vi "OE1311&OE1351_Configure Ref Phase.vi"(7 "OE1300_Configure Ref Phase":T1={"Reference Source"=0, "Internal Frequency(Hz)"=1000.0, "Phase  (degree)"=0.0, "External Ref Trigger"=0, "Instrument Mode "=4} {"Instrument Mode" items=["OE1311"=3, "OE1351"=4, "OE1301"=5]; "External Ref Trigger" items=["TTL Rising Edge", "TTL Fallling Edge", "Sine Zero Crossing"]; "Phase  (degree)" min=-180.0 max=180.0 format="%#.2g"; "Internal Frequency(Hz)" min=0.001 max=1002000.0 format="%#.3f"; "Reference Source" items=["External", "Internal", "Self"]}, 8 "Error in (no error)":errorcluster caption="error out（no error）", 9 "Remote Mode":u16(ring)=1 items=["RS232"=1, "Ethernet"=3], 10 "Connection ID in":refnum<k5>, 11 "VISA resource name":refnum<visa-resource-name>) -> (0 "Error out":errorcluster caption="error out", 1 "Output String":string, 2 "Connection ID out":refnum<k5>, 3 "VISA resource  out":refnum<visa-resource-name>)   [LabVIEW 2011]
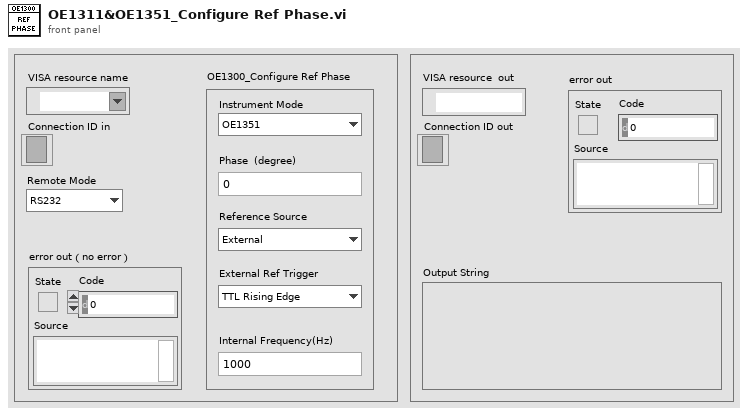
[diagram p1: front panel]
types:
  T1 = cluster{"Reference Source":u16, "Internal Frequency(Hz)":dbl, "Phase  (degree)":dbl, "External Ref Trigger":u16, "Instrument Mode ":u16}
  T2 = enum16{"ISRC", "IGND", "ICPL", "ILIN", "PHAS", "FMOD", "RSLP", "FREQ", "SWPT", "SLLM", "SULM", "SSLL", "SSLG", "STLM", "SWRM", "IRNG", "SENS", "RMOD", "OFLT", "OFSL", "SYNC", "DMOD", "HARM", "DARB", "SWVT", "SLVL", "SVLL", "SVUL", "SVSL", "SVSG", "SVTM", "SVRM", "RALL", "SNAP", "OUTP", "OAUX", "COUT", "CAUX", "COFP", "CEXP", "FPOP", "OEXP", "*IDN", "*RST", "OVLD", "INOV", "GNOV", "*PLL", "SSET", "RSET", "AGAN", "APHS", "ARSV", "ASCL", "EQCD", "EQCS", "SPED", "SRAT", "SLEN", "SSLE", "STRG", "SPRM", "STRD", "PAUS", "REST", "SPTS", "TRCA", "TEMP", "RSTU", "IHNZ", "DEQU", "SADD", "ARNG", "CSPE", "ISRCD", "IGNDD", "ICPLD", "ILIND", "PHASD", "FMODD", "RSLPD", "FREQD", "SWPTD", "SLLMD", "SULMD", "SSLLD", "SSLGD", "STLMD", "SWRMD", "SENSD", "RMODD", "OFLTD", "OFSLD", "SYNCD", "HARMD", "EQCDD", "EQCSD", "SNAPD", "OUTPD", "SWVTD", "SLVLD", "SVLLD", "SVULD", "SVSLD", "SVSGD", "SVTMD", "SVRMD", "SVDCD", "ARSVD", "AGAND", "APHSD", "ASCLD", "FPOPD", "CAUXD", "OEXPD", "SPEDD", "SRATD", "SLEND", "SSLED", "STRGD", "SPRMD", "STRDD", "PAUSD", "RESTD", "SPTSD", "TRCAD", "*IDND", "*RSTD", "INOVD", "GNOVD", "*PLLD", "SSETD", "RSETD", "RALLD"}
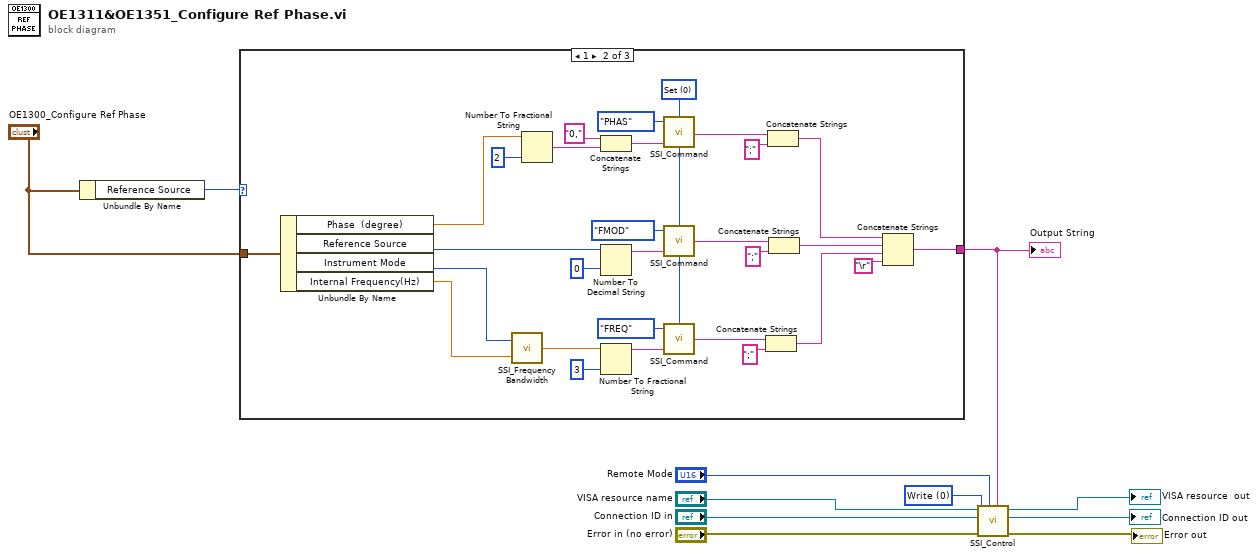
[diagram p0: block diagram]
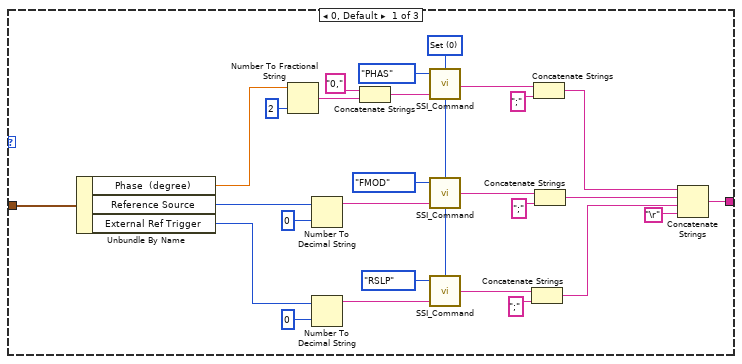
[diagram p2: hidden frame]
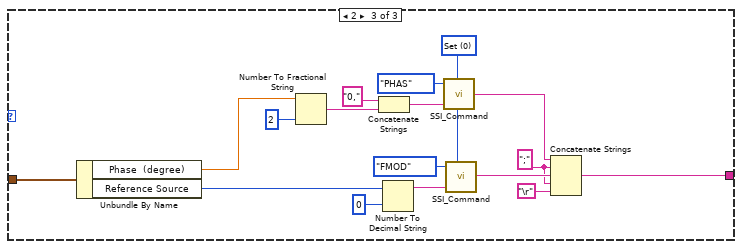
[diagram p3: hidden frame]
diagram:
  w9 = u16 0 items=["Write", "Read"] ("Control")
  n1 = Unbundle By Name("OE1300_Configure Ref Phase") -> ("Reference Source"=w4:u16)
  n2 = case shown="1" w4 {
    tunnel: "OE1300_Configure Ref Phase" -> [w26 w51 w80]
    tunnel: [w20 w50 w77] -> w5
    frame 0, Default {
      w25 = u16 0 items=["Set", "Query"] ("Opera")
      n3 = Unbundle By Name(w26) -> ("Phase  (degree)"=w15:dbl, "Reference Source"=w24:u16, "External Ref Trigger"=w27:u16)
      n4 = Number To Fractional String(number=w15, precision (6)=i16 2 ("精度(6)")) -> (F-format string=w12:string)  [unwired: 2 in]
      n5 = Number To Decimal String(number=w24, width (-)=i16 0 ("精度(6)")) -> (decimal integer string=w36:string)
      n6 = Number To Decimal String(number=w27, width (-)=i16 0 ("精度(6)")) -> (decimal integer string=w34:string)
      n7 = Concatenate Strings("0," ("字符串"), w12) -> (w14:string)
      n8 = call "SSI_Command.vi"("Opera"=w25, "Paramter"=w14, "Command Type"=T2."PHAS") -> ("Output string"=w28:string)  [unwired: 1 in]
      n9 = call "SSI_Command.vi"("Opera"=w25, "Paramter"=w36, "Command Type"=T2."FMOD") -> ("Output string"=w30:string)  [unwired: 1 in]
      n10 = call "SSI_Command.vi"("Opera"=w25, "Paramter"=w34, "Command Type"=T2."RSLP") -> ("Output string"=w33:string)  [unwired: 1 in]
      n11 = Concatenate Strings(w33, ";" ("替换字符串(\"\")")) -> (w21:string)
      n12 = Concatenate Strings(w28, ";" ("替换字符串(\"\")")) -> (w23:string)
      n13 = Concatenate Strings(w30, ";" ("替换字符串(\"\")")) -> (w22:string)
      n14 = Concatenate Strings(w23, w22, w21, "\r") -> (w20:string)
    }
    frame 1 {
      w56 = u16 0 items=["Set", "Query"] ("Opera")
      n15 = Unbundle By Name(w51) -> ("Phase  (degree)"=w46:dbl, "Reference Source"=w55:u16, "Instrument Mode"=w42:u16, "Internal Frequency(Hz)"=w43:dbl)
      n16 = call "SSI_Frequency Bandwidth.vi"("Frequency"=w43, "Instrument Mode"=w42) -> ("Output"=w44:dbl)  [unwired: 1 in]
      n17 = Number To Fractional String(number=w46, precision (6)=i16 2 ("精度(6)")) -> (F-format string=w40:string)  [unwired: 2 in]
      n18 = Concatenate Strings("0," ("字符串"), w40) -> (w39:string)
      n19 = Number To Decimal String(number=w55, width (-)=i16 0 ("精度(6)")) -> (decimal integer string=w65:string)
      n20 = Number To Fractional String(number=w44, precision (6)=i16 3 ("精度(6)")) -> (F-format string=w63:string)  [unwired: 2 in]
      n21 = call "SSI_Command.vi"("Opera"=w56, "Paramter"=w39, "Command Type"=T2."PHAS") -> ("Output string"=w57:string)  [unwired: 1 in]
      n22 = call "SSI_Command.vi"("Opera"=w56, "Paramter"=w65, "Command Type"=T2."FMOD") -> ("Output string"=w59:string)  [unwired: 1 in]
      n23 = call "SSI_Command.vi"("Opera"=w56, "Paramter"=w63, "Command Type"=T2."FREQ") -> ("Output string"=w62:string)  [unwired: 1 in]
      n24 = Concatenate Strings(w62, ";" ("替换字符串(\"\")")) -> (w52:string)
      n25 = Concatenate Strings(w57, ";" ("替换字符串(\"\")")) -> (w54:string)
      n26 = Concatenate Strings(w59, ";" ("替换字符串(\"\")")) -> (w53:string)
      n27 = Concatenate Strings(w54, w53, w52, "\r") -> (w50:string)
    }
    frame 2 {
      w71 = u16 0 items=["Set", "Query"] ("Opera")
      w73 = ";" ("替换字符串(\"\")")
      n28 = Unbundle By Name(w80) -> ("Phase  (degree)"=w72:dbl, "Reference Source"=w81:u16)
      n29 = Number To Fractional String(number=w72, precision (6)=i16 2 ("精度(6)")) -> (F-format string=w69:string)  [unwired: 2 in]
      n30 = Concatenate Strings("0," ("字符串"), w69) -> (w70:string)
      n31 = Number To Decimal String(number=w81, width (-)=i16 0 ("精度(6)")) -> (decimal integer string=w83:string)
      n32 = call "SSI_Command.vi"("Opera"=w71, "Paramter"=w70, "Command Type"=T2."PHAS") -> ("Output string"=w74:string)  [unwired: 1 in]
      n33 = call "SSI_Command.vi"("Opera"=w71, "Paramter"=w83, "Command Type"=T2."FMOD") -> ("Output string"=w82:string)  [unwired: 1 in]
      n34 = Concatenate Strings(w74, w73, w82, w73, "\r") -> (w77:string)
    }
  }
  "Output String" <- w5
  n35 = call "SSI_Control.vi"("Write Buffer"=w5, "Remote Mode"="Remote Mode", "Error in (no error)"="Error in (no error)", "Control"=w9, "Connection ID in"="Connection ID in", "VISA resource name"="VISA resource name") -> ("Error out"=→"Error out":errorcluster, "Connection ID out"=→"Connection ID out":refnum<k5>, "VISA resource  out"=→"VISA resource  out":refnum<visa-resource-name>)  [unwired: 2 in, 1 out]
